vi "sampleIndex_2_NoofSamplesinPSChans.vi"(1 "Sample Index":i32[](array[numeric])) -> (0 "No of Samples in PS Chans":i32)   [LabVIEW 2013]
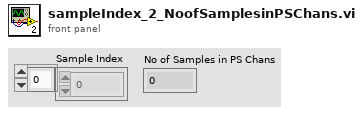
[diagram p1: front panel]
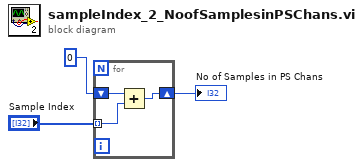
[diagram p0: block diagram]
diagram:
  n1 = for {
    tunnel: "Sample Index" -> [w5] mode=indexing
    shift-right: [w4] -> w1
    shift-left: 0 -> [w6]
    n2 = Add(x=w6, y=w5) -> (x+y=w4:i32)
  }
  "No of Samples in PS Chans" <- w1
